vi "Buffer Initialize.vi"(8 "error in (no error)":errorcluster, 9 "Number Of Elements":i32, 10 "Sector Number":i32, 11 "Circular Buffer 1D U16 DVR Queue in":refnum<class "Circular Buffer 1D U16 DVR Queue.lvclass">) -> (0 "error out":errorcluster, 3 "Circular Buffer 1D U16 DVR Queue out":refnum<class "Circular Buffer 1D U16 DVR Queue.lvclass">)   [LabVIEW 2019, in "Circular Buffer 1D U16 DVR Queue.lvclass"]
uses:
  Circular Buffer 1D U16 DVR Queue.lvclass
  Type Def/1D U16 DVR.ctl
  Circular Buffer 1D U16 DVR Queue.lvclass/Circular Buffer 1D U16 DVR Queue.ctl
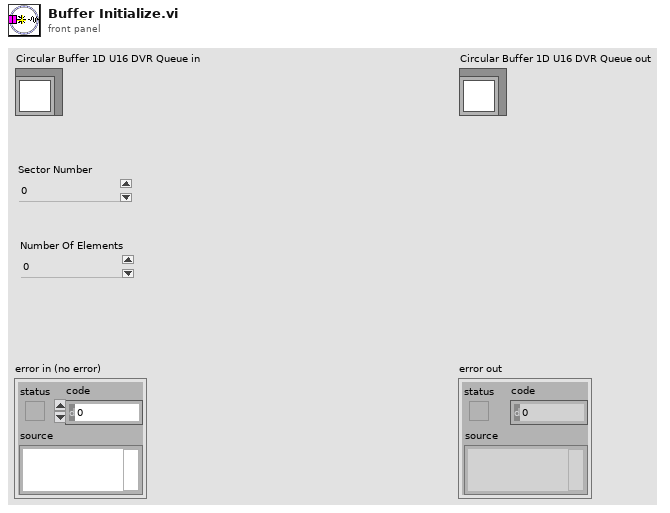
[diagram p1: front panel]
types:
  T1 = typedef "1D U16 DVR.ctl" = refnum<data-value>
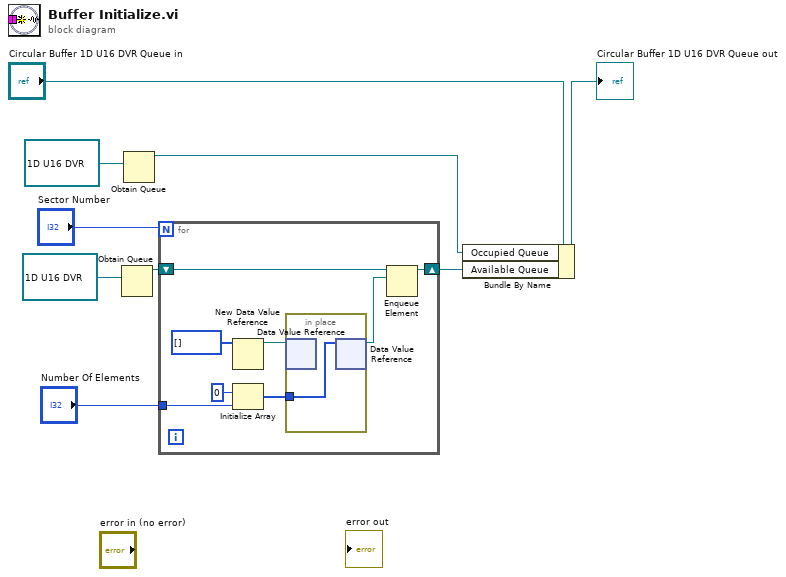
[diagram p0: block diagram]
diagram:
  n1 = Obtain Queue(element data type=T1 refnum ("1D U16 DVR")) -> (queue out=w6:refnum<queue>)  [unwired: 4 in, 2 out]
  n2 = Obtain Queue(element data type=T1 refnum ("1D U16 DVR")) -> (queue out=w2:refnum<queue>)  [unwired: 4 in, 2 out]
  n3 = for {
    N: "Sector Number" -> [_]
    tunnel: "Number Of Elements" -> [w16]
    shift-right: [w10] -> w3
    shift-left: w6 -> [w12]
    n4 = New Data Value Reference(data value=u16[] [] ("initialized array")) -> (data value reference=w14:refnum<data-value>)  [unwired: 1 in, 1 out]
    n5 = Initialize Array(u16 0 ("element"), w16) -> (w13:u16[])
    n6 = in-place {
      in-place-border: w13 -> [w18]
      n7 = in-place-dvr #1(w14) -> ()  [unwired: 2 out]
      n8 = in-place-dvr #1(w18) -> (w11:refnum<data-value>)  [unwired: 1 out]
    }
    n9 = Enqueue Element(queue=w12, element=w11) -> (queue out=w10:refnum<queue>)  [unwired: 2 in, 2 out]
  }
  n10 = Bundle By Name(cluster="Circular Buffer 1D U16 DVR Queue in", "Occupied Queue"=w2, "Available Queue"=w3) -> (→"Circular Buffer 1D U16 DVR Queue out":refnum<class "Circular Buffer 1D U16 DVR Queue.lvclass">)
